vi "UT_003_TOML to LV.vi"() -> ()   [LabVIEW 2017]
uses:
  c9d3ce3a-f03d-491e-936c-17ec64c2196e.vi
  a84c01b4-b6b6-4be3-a592-8d4feadcdc62.vi
  8d36a4aa-f2c5-4afc-9410-2bff02845cb1.vi
  lib/TOML to LabVIEW.vi
  <vilib>/addons/_JKI Toolkits/Caraya/classes/Assert/Assert True.vi
  <vilib>/addons/_JKI Toolkits/Caraya/classes/Test/Test.lvclass
  <vilib>/addons/_JKI Toolkits/Caraya/classes/Assert/Assert.lvclass
  lib/TOML.lvlib
panel:
  out "3":string[](array[string])
  out "2":string[](array[string])
  out "1":string[](array[string])
  out "error out":errorcluster
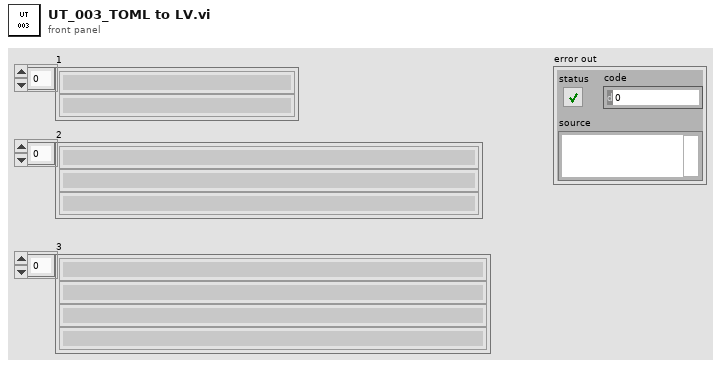
[diagram p1: front panel]
types:
  T1 = cluster{"cluster":cluster{"status":bool, "code":i32, "source":string, "error":errorcluster, "float-array":dbl[], "cluster-array":cluster{"nme":string, "value":dbl}[]}}
  T2 = cluster{"cluster":cluster{"status":bool, "code":i32, "source":string, "error":cluster{"status":bool, "code":i32, "souce":string}, "float-array":dbl[], "cluster-array":cluster{"name":string, "value":dbl}[]}}
  T3 = cluster{"cluster":cluster{"status":bool, "cde":i32, "source":string, "error":errorcluster, "float-array":dbl[], "cluster-array":cluster{"name":string, "value":dbl}[]}}
  T4 = typedef "TOML.lvlib/TOML Value.ctl" = cluster{"type":enum16{"Table", "Array", "String", "Integer", "Float", "Boolean", "Offset Date-Time", "Local Date-Time", "Local Date", "Local Time"}, "value":variant}
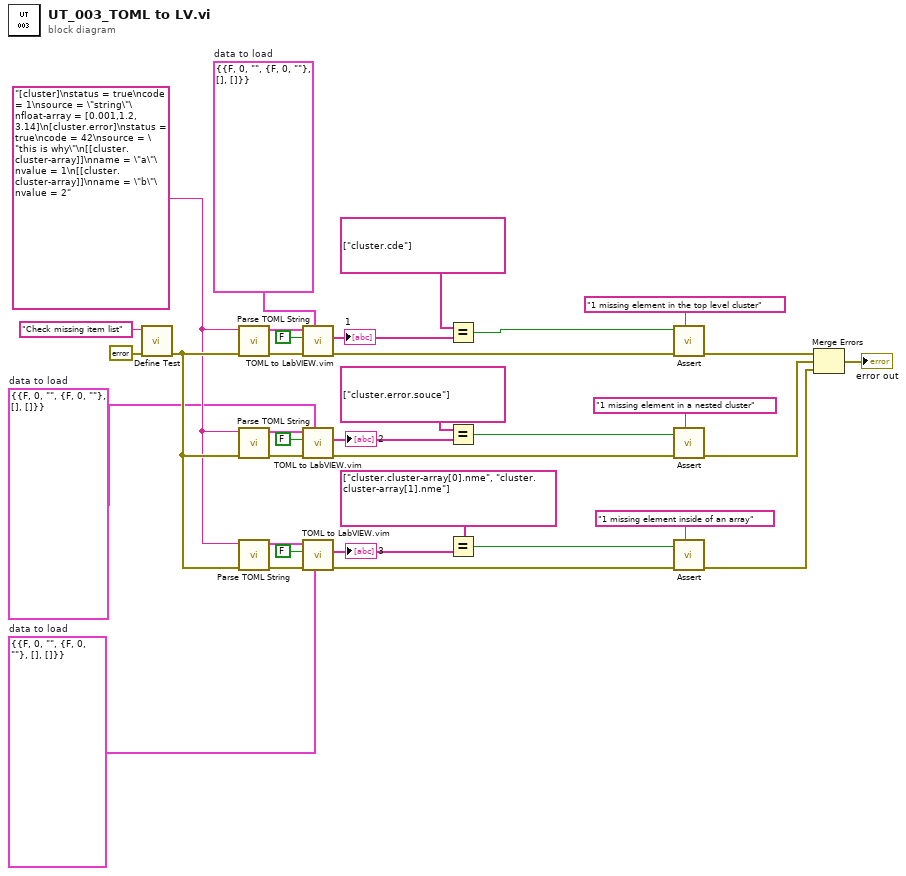
[diagram p0: block diagram]
diagram:
  w1 = T1 {"cluster"={"status"=FALSE, "code"=0, "source"="", "error"={"status"=FALSE, "code"=0, "source"=""}, "float-array"=[], "cluster-array"=[]}}  # data to load
  w6 = T2 {"cluster"={"status"=FALSE, "code"=0, "source"="", "error"={"status"=FALSE, "code"=0, "souce"=""}, "float-array"=[], "cluster-array"=[]}}  # data to load
  w13 = T3 {"cluster"={"status"=FALSE, "cde"=0, "source"="", "error"={"status"=FALSE, "code"=0, "source"=""}, "float-array"=[], "cluster-array"=[]}}  # data to load
  w20 = "[cluster]\nstatus = true\ncode = 1\nsource = \"string\"\nfloat-array = [0.001,1.2, 3.14]\n[cluster.error]\nstatus = true\ncode = 42\nsource = \"this is why\"\n[[cluster.cluster-array]]\nname = \"a\"\nvalue = 1\n[[cluster.cluster-array]]\nname = \"b\"\nvalue = 2" ("String")
  n1 = call <vilib>:"Define Test.vi"("error in (no error)"=errorcluster {"status"=FALSE, "code"=0, "source"=""}, "Label (VI Title)"="Check missing item list") -> ("error out"=w21:errorcluster)  [unwired: 9 in]
  n2 = call "Parse TOML String.vi"("error in (no error)"=w21, "String"=w20) -> ("error out"=w17:errorcluster, "Value"=w18:T4)  [unwired: 8 in]
  n3 = call "Parse TOML String.vi"("error in (no error)"=w21, "String"=w20) -> ("error out"=w10:errorcluster, "Value"=w12:T4)  [unwired: 8 in]
  n4 = call "Parse TOML String.vi"("error in (no error)"=w21, "String"=w20) -> ("error out"=w3:errorcluster, "Value"=w7:T4)  [unwired: 8 in]
  n5 = call "TOML to LabVIEW.vim"("datatype"=w13, "error in (no error)"=w17, "Error if missing element"=FALSE, "Value"=w18) -> ("error out"=w16:errorcluster, "Missing elements"=w15:string[])  [unwired: 5 in, 1 out]
  "1" <- w15
  n6 = call "TOML to LabVIEW.vim"("datatype"=w6, "error in (no error)"=w10, "Error if missing element"=FALSE, "Value"=w12) -> ("error out"=w9:errorcluster, "Missing elements"=w8:string[])  [unwired: 5 in, 1 out]
  "2" <- w8
  n7 = call "TOML to LabVIEW.vim"("datatype"=w1, "error in (no error)"=w3, "Error if missing element"=FALSE, "Value"=w7) -> ("error out"=w2:errorcluster, "Missing elements"=w5:string[])  [unwired: 5 in, 1 out]
  "3" <- w5
  n8 = Equal?(x=string[] ["cluster.cde"], y=w15) -> (x = y?=w28:bool)
  n9 = Equal?(x=string[] ["cluster.error.souce"], y=w8) -> (x = y?=w27:bool)
  n10 = Equal?(x=string[] ["cluster.cluster-array[0].nme", "cluster.cluster-array[1].nme"], y=w5) -> (x = y?=w23:bool)
  n11 = call-poly <vilib>:"Assert.vi"("Label"="1 missing element in the top level cluster" ("Label (VI Title)"), "error in (no error)"=w16, "True?"=w28) -> ("error out"=w34:errorcluster)  [unwired: 8 in]
  n12 = call-poly <vilib>:"Assert.vi"("Label"="1 missing element in a nested cluster" ("Label (VI Title)"), "error in (no error)"=w9, "True?"=w27) -> ("error out"=w29:errorcluster)  [unwired: 8 in]
  n13 = call-poly <vilib>:"Assert.vi"("Label"="1 missing element inside of an array" ("Label (VI Title)"), "error in (no error)"=w2, "True?"=w23) -> ("error out"=w19:errorcluster)  [unwired: 8 in]
  n14 = Merge Errors(w34, w29, w19) -> (→"error out":errorcluster)
